vi "Map_setCursorPosition.vi"(1 "cursor position":cluster{"X":sgl, "Y":sgl}, 2 "existing\ncursor name":string="poly", 3 "graph ref":refnum<vi>) -> ()   [LabVIEW 2010]
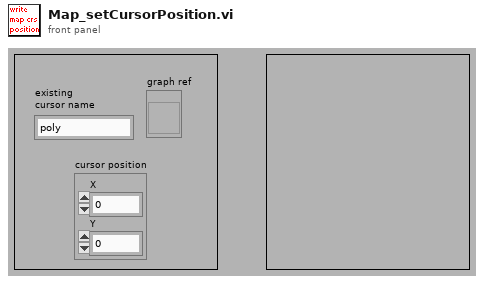
[diagram p1: front panel]
types:
  T1 = typedef "LVCursorListTypeDef.ctl" = cluster{"Name":string, "Color":u32, "Style":u8, "Point Style":u8, "Name Visible":bool, "Allow Drag":bool, "Cursor Mode":u32, "Plot":i32, "Index":i32, "Position":cluster{"X":dbl, "Y":dbl}, "X Scale":u32, "Y Scale":u32, "Watch Plots":i32[], "Watch All Plots":bool, "Plot Area":i32, "Label Offset":cluster{"X":dbl, "Y":dbl}}[]
  T2 = cluster{"Name":string, "Color":u32, "Style":u8, "Point Style":u8, "Name Visible":bool, "Allow Drag":bool, "Cursor Mode":u32, "Plot":i32, "Index":i32, "Position":cluster{"X":dbl, "Y":dbl}, "X Scale":u32, "Y Scale":u32, "Watch Plots":i32[], "Watch All Plots":bool, "Plot Area":i32, "Label Offset":cluster{"X":dbl, "Y":dbl}}
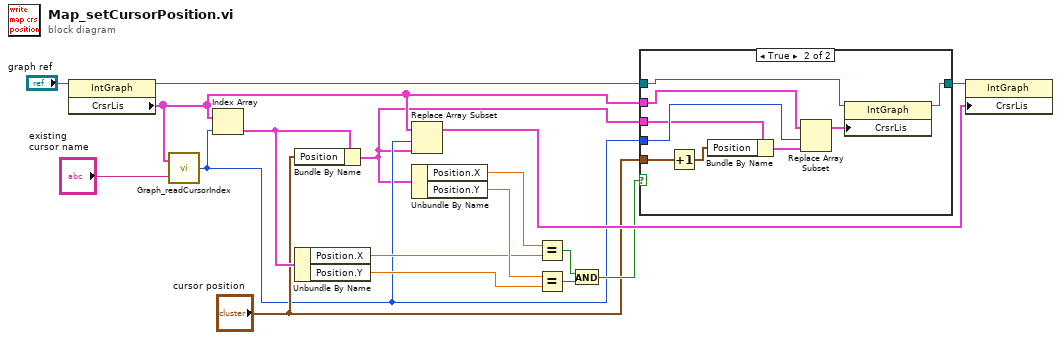
[diagram p0: block diagram]
diagram:
  n1 = property class="IntGraph"(reference="graph ref") -> (reference out=w5:refnum<vi>, "CrsrLis"=w4:T1)  [unwired: 1 in, 1 out]
  n2 = call "Graph_readCursorIndex.vi"("existing cursor\nname"="existing\ncursor name", "Cursor List"=w4) -> ("cursor index"=w2:i32)
  n3 = Index Array(array=w4, index=w2) -> (element=w14:T2)
  n4 = Bundle By Name(cluster=w14, "Position"="cursor position") -> (w1:T2)
  n5 = Unbundle By Name(w14) -> ("Position.X"=w11:dbl, "Position.Y"=w13:dbl)
  n6 = Replace Array Subset(array=w4, new element=w1, index=w2) -> (w15:T1)
  n7 = Unbundle By Name(w1) -> ("Position.X"=w10:dbl, "Position.Y"=w12:dbl)
  n8 = Equal?(x=w10, y=w11) -> (x = y?=w9:bool)
  n9 = Equal?(x=w12, y=w13) -> (x = y?=w8:bool)
  n10 = And(x=w9, y=w8) -> (x .and. y?=w7:bool)
  n11 = case shown="True" w7 {
    tunnel: w1 -> [_ w22]
    tunnel: w2 -> [_ w27]
    tunnel: [w18 w19] -> w6
    tunnel: w5 -> [w18 w20]
    tunnel: w4 -> [_ w26]
    tunnel: "cursor position" -> [_ w24]
    frame False {
    }
    frame True {
      n12 = Increment(x=w24) -> (x+1=w23:cluster{"X":sgl, "Y":sgl})
      n13 = Bundle By Name(cluster=w22, "Position"=w23) -> (w21:T2)
      n14 = Replace Array Subset(array=w26, new element=w21, index=w27) -> (w25:T1)
      n15 = property class="IntGraph"(reference=w20, "CrsrLis"=w25) -> (reference out=w19:refnum<vi>)  [unwired: 1 in, 1 out]
    }
  }
  n16 = property class="IntGraph"(reference=w6, "CrsrLis"=w15) -> ()  [unwired: 1 in, 2 out]
